vi "Begin.vi"(8 "error in":errorcluster) -> (0 "error out":errorcluster)   [LabVIEW 2014]
doc: "Called before other user functions, this VI is expected to open initial I/O refnums, load in file data, and do all program initialization. Notice that the <B>error out</B> terminal is simply used for data flow. Wiring it to other structures or subVIs ensures that this VI runs first."
uses:
  <vilib>/Rock Robotics/SystemInterfaces/DIO/FPGA_DIOPWMChannel.ctl
  <vilib>/Rock Robotics/WPI/SafetyOutput/WPI_SafetyOutputConfigMenu.ctl
  <vilib>/Rock Robotics/WPI/DriverStation/WPI_DriverStationRobotMode2.ctl
  <vilib>/Rock Robotics/WPI/Joystick/WPI_JoystickDeviceEnum.ctl
  <vilib>/Rock Robotics/SystemInterfaces/DIO/FPGA_DIOChannel.ctl
  <vilib>/Rock Robotics/SystemInterfaces/AI/FPGA_AIGyroChannel.ctl
  <vilib>/Rock Robotics/SystemInterfaces/AI/FPGA_AIChannel.ctl
  <vilib>/Rock Robotics/WPI/RobotDrive/WPI_RobotDriveOpen2MotorWithTalon.vi
  Robot Global Data.vi
  <vilib>/Rock Robotics/Network Tables/SD Write String Array.vi
  <vilib>/Rock Robotics/WPI/Counter/WPI_CounterDigitalInputToDigitalSource.vi
  <vilib>/Rock Robotics/WPI/MotorControl/WPI_MotorControlOpen Talon.vi
  <vilib>/Rock Robotics/WPI/Ultrasonic/WPI_SonarMB1010AnalogOpen.vi
  <vilib>/Rock Robotics/WPI/Ultrasonic/WPI_SonarMB1010AnalogRefNum Registry Set.vi
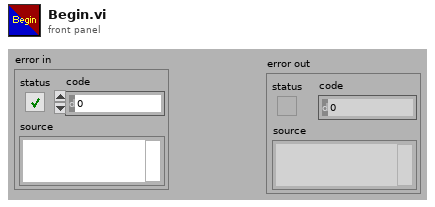
[diagram p1: front panel]
types:
  T1 = typedef "FPGA_DIOChannel.ctl" = enum8{"DIO 0", "DIO 1", "DIO 2", "DIO 3", "DIO 4", "DIO 5", "DIO 6", "DIO 7", "DIO 8", "DIO 9", "DIO MXP 0", "DIO MXP 1", "DIO MXP 2", "DIO MXP 3", "DIO MXP 4", "DIO MXP 5", "DIO MXP 6", "DIO MXP 7", "DIO MXP 8", "DIO MXP 9", "DIO MXP 10", "DIO MXP 11", "DIO MXP 12", "DIO MXP 13", "DIO MXP 14", "DIO MXP 15", "Invalid"}
  T2 = typedef "FPGA_DIOPWMChannel.ctl" = enum8{"PWM 0", "PWM 1", "PWM 2", "PWM 3", "PWM 4", "PWM 5", "PWM 6", "PWM 7", "PWM 8", "PWM 9", "PWM MXP 0", "PWM MXP 1", "PWM MXP 2", "PWM MXP 3", "PWM MXP 4", "PWM MXP 5", "PWM MXP 6", "PWM MXP 7", "PWM MXP 8", "PWM MXP 9", "Invalid"}
  T3 = typedef "FPGA_AIChannel.ctl" = enum8{"AI 0", "AI 1", "AI 2", "AI 3", "AI MXP 0", "AI MXP 1", "AI MXP 2", "AI MXP 3", "Invalid"}
  T4 = typedef "FPGA_AIGyroChannel.ctl" = enum8{"AI 0", "AI 1", "Invalid"}
  T5 = typedef "WPI_JoystickDeviceEnum.ctl" = enum16{"USB 0", "USB 1", "USB 2", "USB 3", "USB 4", "USB 5"}
  T6 = typedef "WPI_DriverStationRobotMode2.ctl" = enum16{"Autonomous Disabled", "Autonomous Enabled", "Teleop Disabled", "Teleop Enabled", "Disconnected", "Finish", "Test Disabled", "Test Enabled", "Emergency Stopped"}
  T7 = typedef "WPI_SafetyOutputConfigMenu.ctl" = enum16{"Enable", "Disable"}
  T8 = typedef "WPI_CompressorDevRef.ctl" = cluster{"DevStatus":errorcluster, "Pneumatics Control Module":u8}
  T9 = typedef "WPI_JoystickDevRef.ctl" = cluster{"Device":T5}
  T10 = typedef "WPI_RobotDriveDevRef.ctl" = cluster{"DevStatus":errorcluster, "Motors[]":T11[], "Square Inputs":bool, "Max Output":dbl}
  T11 = typedef "WPI_MotorControlDeviceRef.ctl" = cluster{"DeviceStatus":errorcluster, "Type":T12, "PWM":cluster{"Controller":T13, "PWM Channel":T2, "DeadBand":T14}, "CAN":cluster{"Device Number":u8, "Control Mode":T15, "Semaphore":T16, "Max Vout":dbl, "TalonSRX Control Mode":T17}, "Invert":bool, "TransformRef":T18, "InvTransformRef":T18}
  T12 = typedef "WPI_MotorControlType.ctl" = enum16{"PWM", "CAN", "CANTalonSRX"}
  T13 = typedef "FPGA_TypedefDigitalModule.ctl" = enum16{"Controller 1"}
  T14 = typedef "WPI_PWMDeadband.ctl" = cluster{"Name":string, "maxPositivePwm":i32, "minPositivePwm":i32, "centerPwm":i32, "maxNegativePwm":i32, "minNegativePwm":i32, "angularRange":u16}
  T15 = typedef "WPI_CANJaguar_ControlMode.ctl" = enum8{"Percent VBus", "Current", "Speed", "Position", "Voltage"}
  T16 = typedef "Semaphore RefNum" = refnum<k1>
  T17 = typedef "WPI_CANTalonSRX_APIControlMode.ctl" = enum8{"Percent VBus", "Speed", "Position", "Slave", "Unchanged / Invalid"}
  T18 = typedef "WPI_PWMTransform_ConPane.ctl" = refnum<vi>
  T19 = typedef "WPI_DigitalInputDevRef.ctl" = cluster{"DevStatus":errorcluster, "DIO Channel":T1, "Controller":T13}
  T20 = typedef "FPGA_CounterEncoderSourceConvertionLVSourceType.ctl" = cluster{"DevStatus":errorcluster, "AnalogTriggerMode?":bool, "DigitalMode":cluster{"Controller":T13, "DIO Channel":T21}, "AnalogTriggerMode":cluster{"AnalogTriggerIndex":T22, "OutputType":T23}}
  T21 = typedef "FPGA_DIODigitalSourceChannel.ctl" = enum8{"DIO 0", "DIO 1", "DIO 2", "DIO 3", "DIO 4", "DIO 5", "DIO 6", "DIO 7", "DIO 8", "DIO 9", "DIO MXP 0", "DIO MXP 1", "DIO MXP 2", "DIO MXP 3", "DIO MXP 4", "DIO MXP 5", "DIO MXP 6", "DIO MXP 7", "DIO MXP 8", "DIO MXP 9", "DIO MXP 10", "DIO MXP 11", "DIO MXP 12", "DIO MXP 13", "DIO MXP 14", "DIO MXP 15", "Disabled"}
  T22 = typedef "FPGA_AnalogTriggerIndex.ctl" = enum8{"Trig 0", "Trig 1", "Trig 2", "Trig 3", "Trig 4", "Trig 5", "Trig 6", "Trig 7", "Invalid"}
  T23 = typedef "FPGA_AnalogTriggerOutType.ctl" = enum16{"InWindow", "TriggerState", "Rising", "Falling"}
  T24 = typedef "WPI_SonarMB1010AnalogDeviceRef.ctl" = cluster{"AIDeviceRef":T25, "Scaling factor (V/in)":dbl, "Average Bits":u8}
  T25 = typedef "WPI_AnalogChannelDevRef.ctl" = cluster{"DevStatus":errorcluster, "Controller":T26, "Analog Channel":T3}
  T26 = typedef "FPGA_TypedefAnalogModule.ctl" = enum16{"Controller 1"}
  T27 = typedef "WPI_EncoderDevRef.ctl" = cluster{"DevStatus":errorcluster, "EncoderIndex":T28, "CounterIndex":T29, "DistancePerCount":dbl, "Decoding Type":T30}
  T28 = typedef "FPGA_EncoderIdx.ctl" = enum8{"Enc 0", "Enc 1", "Enc 2", "Enc 3", "Enc 4", "Enc 5", "Enc 6", "Enc 7", "Invalid"}
  T29 = typedef "FPGA_CounterCtrSystemIndex.ctl" = enum8{"Ctr 0", "Ctr 1", "Ctr 2", "Ctr 3", "Ctr 4", "Ctr 5", "Ctr 6", "Ctr 7", "Invalid"}
  T30 = typedef "WPI_EncoderType.ctl" = enum16{"1x", "2x", "4x"}
  T31 = typedef "WPI_GyroDevRef.ctl" = cluster{"DevStatus":errorcluster, "Analog Module":T26, "Analog Channel":T3, "Offset":dbl, "Gain (VoltsPerDegree/Second)":dbl}
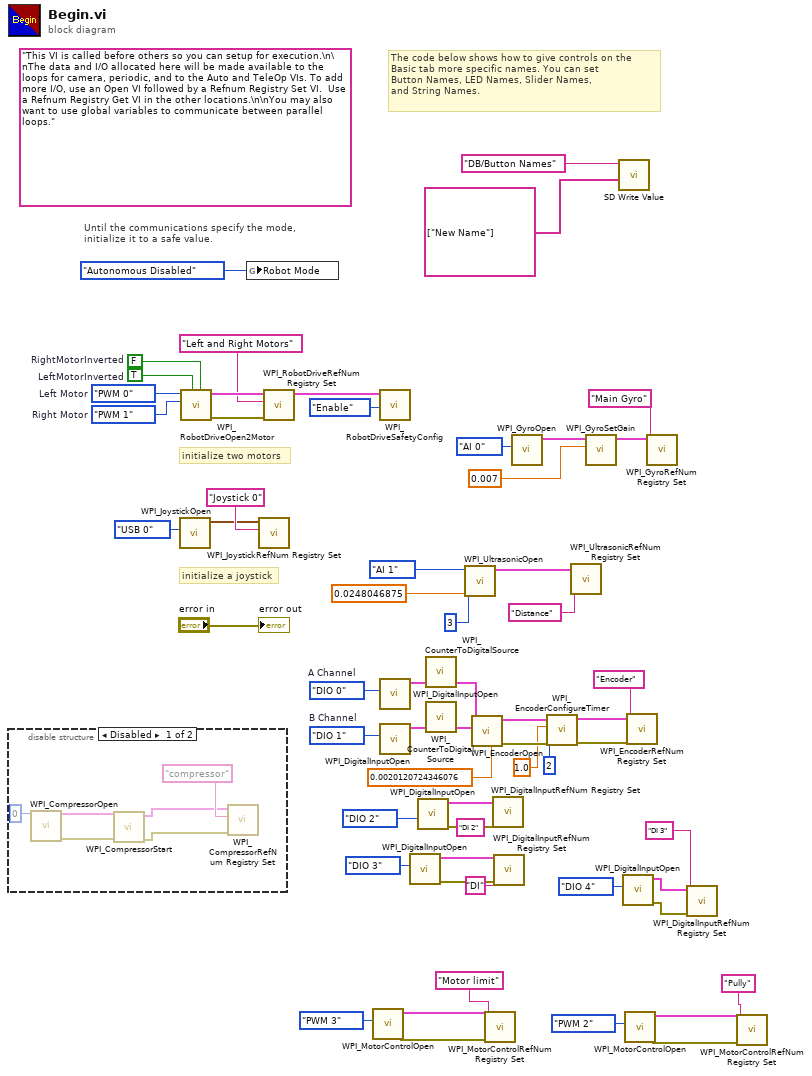
[diagram p0: block diagram]
diagram:
  w44 = FPGA_DIOChannel."DIO 1"  # B Channel
  w43 = FPGA_DIOChannel."DIO 0"  # A Channel
  (unwired) "This VI is called before others so you can setup for execution.\n\nThe data and I/O allocated here will be made available to the loops for camera, periodic, and to the Auto and TeleOp VIs. To add more I/O, use an Open VI followed by a Refnum Registry Set VI.  Use a Refnum Registry Get VI in the other locations.\n\nYou may also want to use global variables to communicate between parallel loops."
  w54 = FPGA_DIOPWMChannel."PWM 1"  # Right Motor
  w55 = FPGA_DIOPWMChannel."PWM 0"  # Left Motor
  w59 = TRUE  # LeftMotorInverted
  w60 = FALSE  # RightMotorInverted
  # "The code below shows how to give controls on the\nBasic tab more specific names. You can set\nButton Names, LED Names, Slider Names,\nand String Names."
  # "initialize a joystick"
  # "Until the communications specify the mode,\ninitialize it to a safe value."
  # "initialize two motors"
  n1 = disable-structure shown="Disabled" {
    frame Disabled {
      n2 = call <vilib>:"WPI_CompressorOpen.vi"("Pneumatics Control Module (0)"=u8 0) -> ("CompressorDevRef"=w65:T8, "error out"=w64:errorcluster)  [unwired: 13 in]
      n3 = call <vilib>:"WPI_CompressorStart.vi"("error in (no error)"=w64, "CompressorDevRef"=w65) -> ("error out"=w62:errorcluster, "CompressorDevRef"=w63:T8)  [unwired: 8 in]
      n4 = call <vilib>:"WPI_CompressorRefNum Registry Set.vi"("error in (no error)"=w62, "refnum name"="compressor", "CompressorDevRef"=w63) -> ()  [unwired: 7 in, 2 out]
    }
    frame Enabled {
    }
  }
  n5 = call <vilib>:"WPI_JoystickOpen.vi"("JoystickDevice"=WPI_JoystickDeviceEnum."USB 0") -> ("JoystickDevRef"=w49:T9)  [unwired: 10 in]
  n6 = call-poly <vilib>:"WPI_RobotDriveOpen2Motor.vi"("Right Motor Inverted"=w60, "Left Motor Inverted"=w59, "Right Motor"=w54, "Left Motor"=w55) -> ("error out"=w56:errorcluster, "RobotDriveDevRef"=w58:T10)  [unwired: 1 in, 5 out]
  n7 = global write "Robot Global Data.vi" "Robot Mode"(WPI_DriverStationRobotMode2."Autonomous Disabled" ("Robot Mode")) -> ()
  n8 = call <vilib>:"WPI_JoystickRefNum Registry Set.vi"("refnum name"="Joystick 0", "JoystickDevRef"=w49) -> ()  [unwired: 8 in, 2 out]
  n9 = call <vilib>:"WPI_RobotDriveRefNum Registry Set.vi"("error in (no error)"=w56, "refnum name"="Left and Right Motors", "RobotDriveDevRef"=w58) -> ("RobotDriveDevRef"=w53:T10)  [unwired: 8 out]
  n10 = call-poly <vilib>:"WPI_MotorControlOpen.vi"("PWM Channel"=FPGA_DIOPWMChannel."PWM 3") -> ("error out"=w17:errorcluster, "MotorControlDeviceRef"=w16:T11)  [unwired: 9 in]
  n11 = call <vilib>:"WPI_RobotDriveSafetyConfig.vi"("mode"=WPI_SafetyOutputConfigMenu."Enable", "RobotDriveDevRef"=w53) -> ()  [unwired: 8 in, 2 out]
  n12 = call <vilib>:"WPI_DigitalInputOpen.vi"("DIO Channel"=w43) -> ("DigitalInputDevRef"=w40:T19)  [unwired: 2 in, 8 out]
  n13 = call <vilib>:"WPI_DigitalInputOpen.vi"("DIO Channel"=w44) -> ("DigitalInputDevRef"=w41:T19)  [unwired: 2 in, 8 out]
  n14 = call <vilib>:"WPI_DigitalInputOpen.vi"("DIO Channel"=FPGA_DIOChannel."DIO 3") -> ("error out"=w7:errorcluster, "DigitalInputDevRef"=w9:T19)  [unwired: 9 in]
  n15 = call <vilib>:"WPI_DigitalInputOpen.vi"("DIO Channel"=FPGA_DIOChannel."DIO 2") -> ("error out"=w8:errorcluster, "DigitalInputDevRef"=w10:T19)  [unwired: 9 in]
  n16 = call-poly <vilib>:"WPI_CounterToDigitalSource.vi"("DigitalInputDevRef"=w40) -> ("Digital Source"=w39:T20)  [unwired: 6 out]
  n17 = call-poly <vilib>:"WPI_CounterToDigitalSource.vi"("DigitalInputDevRef"=w41) -> ("Digital Source"=w42:T20)  [unwired: 6 out]
  n18 = call-poly <vilib>:"WPI_UltrasonicOpen.vi"("Average Bits"=u8 3, "Scaling factor (V/in)"=0.0248046875, "Analog Channel"=FPGA_AIChannel."AI 1") -> ("SonarMB1010AnalogDevRef"=w20:T24)  [unwired: 7 in, 1 out]
  n19 = call <vilib>:"WPI_EncoderOpen.vi"("DistancePerCount"=0.0020120724346076, "BSource"=w42, "ASource"=w39) -> ("error out"=w37:errorcluster, "EncoderDevRef"=w38:T27)  [unwired: 5 in, 2 out]
  n20 = call <vilib>:"WPI_MotorControlRefNum Registry Set.vi"("error in (no error)"=w17, "refnum name"="Motor limit", "MotorControlDevRef"=w16) -> ()  [unwired: 7 in, 2 out]
  n21 = call <vilib>:"WPI_DigitalInputRefNum Registry Set.vi"("error in (no error)"=w8, "refnum name"="DI 2", "DigitalInputDevRef"=w10) -> ()  [unwired: 7 in, 2 out]
  n22 = call <vilib>:"WPI_DigitalInputRefNum Registry Set.vi"("error in (no error)"=w7, "refnum name"="DI", "DigitalInputDevRef"=w9) -> ()  [unwired: 7 in, 2 out]
  n23 = call <vilib>:"WPI_GyroOpen.vi"("Analog Channel"=FPGA_AIGyroChannel."AI 0") -> ("GyroDevRef"=w30:T31)  [unwired: 8 in, 2 out]
  n24 = call <vilib>:"WPI_EncoderConfigureTimer.vi"("error in (no error)"=w37, "Number Samples to Average"=u8 2, "Minimum Rate"=1.0, "EncoderDevRef"=w38) -> ("error out"=w33:errorcluster, "EncoderDevRef"=w34:T27)  [unwired: 6 in]
  n25 = call-poly <vilib>:"WPI_UltrasonicRefNum Registry Set.vi"("refnum name"="Distance", "SonarMB1010AnalogDevRef"=w20) -> ()  [unwired: 8 in, 2 out]
  n26 = call <vilib>:"WPI_GyroSetGain.vi"("Gain (VoltsPerDegree/Second)"=0.007, "GyroDevRef"=w30) -> ("GyroDevRef"=w28:T31)  [unwired: 8 in, 1 out]
  n27 = call-poly <vilib>:"SD Write Value.vi"("String Array"=string[] ["New Name"], "Name"="DB/Button Names") -> ()  [unwired: 8 in, 2 out]
  n28 = call <vilib>:"WPI_DigitalInputOpen.vi"("DIO Channel"=FPGA_DIOChannel."DIO 4") -> ("error out"=w2:errorcluster, "DigitalInputDevRef"=w3:T19)  [unwired: 9 in]
  n29 = call-poly <vilib>:"WPI_MotorControlOpen.vi"("PWM Channel"=FPGA_DIOPWMChannel."PWM 2") -> ("error out"=w26:errorcluster, "MotorControlDeviceRef"=w25:T11)  [unwired: 9 in]
  n30 = call <vilib>:"WPI_EncoderRefNum Registry Set.vi"("error in (no error)"=w33, "refnum name"="Encoder", "EncoderDevRef"=w34) -> ()  [unwired: 7 in, 2 out]
  n31 = call <vilib>:"WPI_GyroRefNum Registry Set.vi"("refnum name"="Main Gyro", "GyroDevRef"=w28) -> ()  [unwired: 8 in, 2 out]
  n32 = call <vilib>:"WPI_DigitalInputRefNum Registry Set.vi"("error in (no error)"=w2, "refnum name"="DI 3", "DigitalInputDevRef"=w3) -> ()  [unwired: 7 in, 2 out]
  n33 = call <vilib>:"WPI_MotorControlRefNum Registry Set.vi"("error in (no error)"=w26, "refnum name"="Pully", "MotorControlDevRef"=w25) -> ()  [unwired: 7 in, 2 out]
  "error out" <- "error in"
